vi "HDF5_Init_TC_Refs.vi"(5 "HDF5 file ref":T1 format="%.0x", 9 "File Exists?":bool, 11 "error in":errorcluster) -> (4 "TC_Refs":T2 {"TC13_Tamb_Inter" format="%.0x"; "TC12_Gen_Exhaust" format="%.0x"; "TC11_HVAC_Cond_Out" format="%.0x"; "TC10_HVAC_Cond_In" format="%.0x"; "TC9_LP2_Lo" format="%.0x"; "TC8_LP2_LoMid" format="%.0x"; "TC7_LP2_Mid" format="%.0x"; "TC6_LP2_MidHi" format="%.0x"; "TC5_LP2_Hi" format="%.0x"; "TC4_LP1_Lo" format="%.0x"; "TC3_LP1_LoMid" format="%.0x"; "TC2_LP1_Mid" format="%.0x"; "TC1_LP1_MidHi" format="%.0x"; "TC0_LP1_Hi" format="%.0x"; "TimeString_dset" format="%.0x"; "TimeStamp_dset" format="%.0x"; "Group_ref" format="%.0x"}, 6 "HDF5 file ref":T1 format="%.0x", 15 "error out":errorcluster)   [LabVIEW 2018]
doc: "Set up the HDF5 data structure and initialize the references for the Tone1, Tone2, Tone3, and Tone4 Groups and the datasets (tables) within each Group.\n\nData structure:\nTone1 (Group) \n Beac - cluster (Dataset)\n BeacZoom - 1024 element Double array (waveform) \n Cal - cluster\n CalZoom - 1024 element Double array (waveform) \nTone2\n Beac - cluster\n BeacZoom - 1024 element Double array (waveform) \n Cal - cluster\n CalZoom - 1024 element Double array (waveform) \nTone3\n Beac - cluster\n BeacZoom - 1024 element Double array (waveform) \n Cal - cluster\n CalZoom - 1024 element Double array (waveform) \nTone4\n Beac - cluster\n BeacZoom - 1024 element Double array (waveform) \n Cal - cluster\n CalZoom - 1024 element Double array (waveform)"
uses:
  <vilib>/addons/h5labview2/base/hid_t.ctl
  TC_Tone_refs.ctl
  lib_path_mod_20200519.vi
  <vilib>/addons/h5labview2/base/H5Equery.vi
  <vilib>/addons/h5labview2/attrib/H5Awrite.llb/H5Awrite.xnode
  <vilib>/addons/h5labview2/group/H5G.lvlib
  <vilib>/addons/h5labview2/dataset/H5D.lvlib
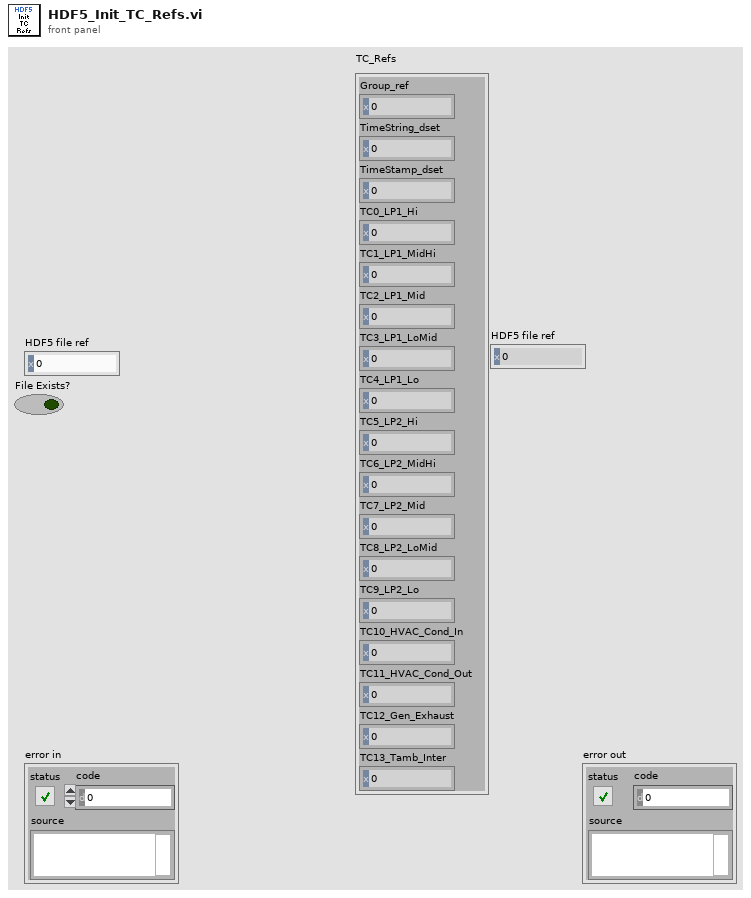
[diagram p1: front panel]
types:
  T1 = typedef "hid_t.ctl" = i32
  T2 = typedef "TC_Tone_refs.ctl" = cluster{"Group_ref":T1, "TimeString_dset":T1, "TimeStamp_dset":T1, "TC0_LP1_Hi":T1, "TC1_LP1_MidHi":T1, "TC2_LP1_Mid":T1, "TC3_LP1_LoMid":T1, "TC4_LP1_Lo":T1, "TC5_LP2_Hi":T1, "TC6_LP2_MidHi":T1, "TC7_LP2_Mid":T1, "TC8_LP2_LoMid":T1, "TC9_LP2_Lo":T1, "TC10_HVAC_Cond_In":T1, "TC11_HVAC_Cond_Out":T1, "TC12_Gen_Exhaust":T1, "TC13_Tamb_Inter":T1}
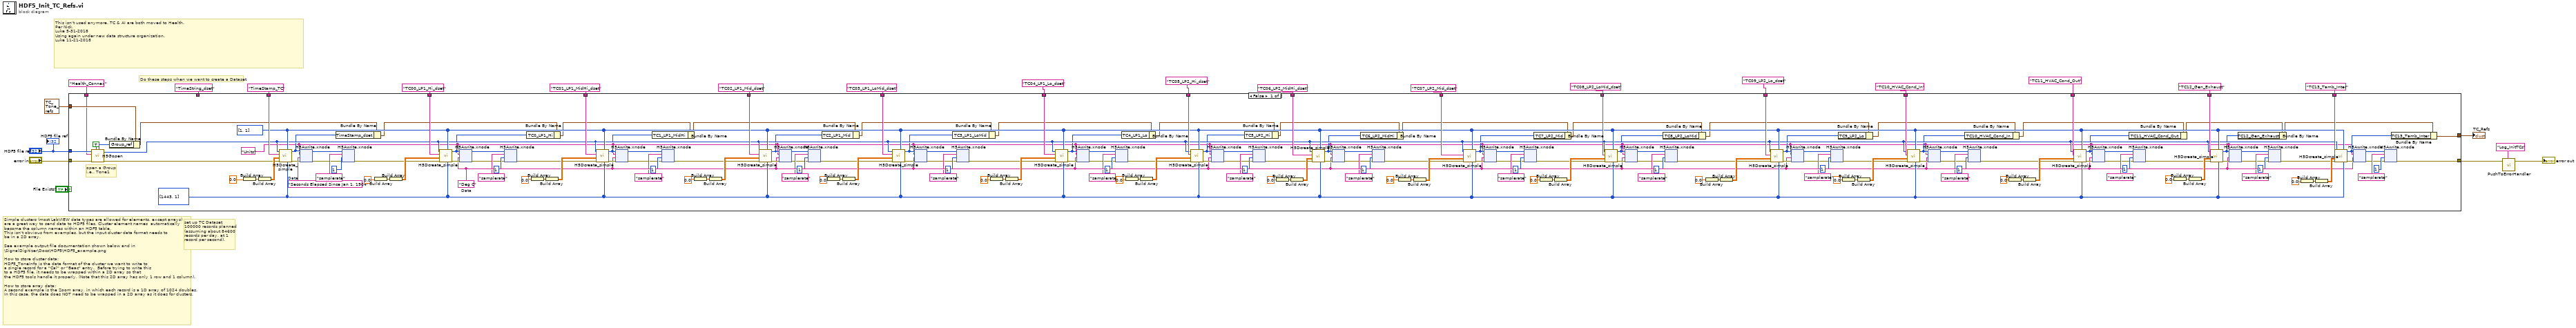
[diagram p0: block diagram]
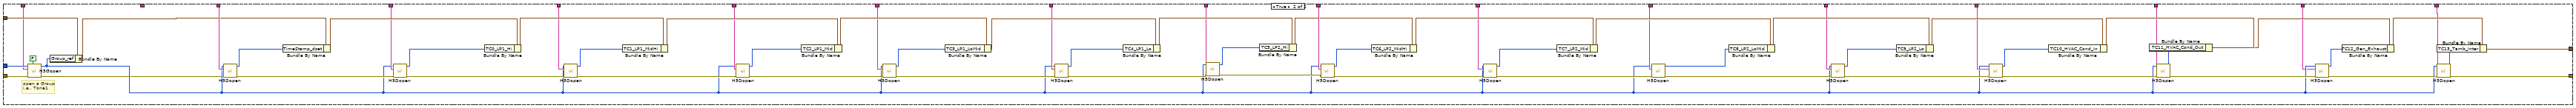
[diagram p2: hidden frame]
diagram:
  # "This isn't used anymore. TC & AI are both moved to Health.\nPer Nick.\nLuke 5-31-2018\nUsing again under new data structure organization.\nLuke 11-21-2018"
  # "Do these steps when we want to create a Dataset"
  # "set up TC Dataset\n100000 records planned\n(assuming about 84600\nrecords per day, at 1\nrecord per second)."
  # "Simple clusters (most LabVIEW data types are allowed for elements, except arrays) \nare a great way to send data to HDF5 files. Cluster element names  automatically\nbecome the column names within an HDF5 table.\nThis isn't obvious from examples, but the input cluster data format needs to \nbe in a 2D array.\n\nSee example output file documentation shown below and in\n\\SignalDigitizer\\Docs\\HDF5\\HDF5_example.png\n\nHow to store cluster data:\nHDF5_ToneInfo is the data format of the cluster we want to write to \na single record for a \"Cal\" or \"Beac\" entry.  Before trying to write this \nto a HDF5 file, it needs to be wrapped within a 2D array so that \nthe HDF5 tools handle it properly. (Note that this 2D array has only 1 row and 1 column).\n\nHow to store array data:\nA second example is the Zoom array, in which each record is a 1D array of 1024 doubles.\nIn this case, the data does NOT need to be wrapped in a 2D array as it does for clusters."
  n1 = case shown="False" "File Exists?" {
    tunnel: "error in" -> [w218 w856]
    tunnel: "HDF5 file ref" -> [w217 w855]
    tunnel: [w27 w792] -> w2
    tunnel: T2 {"Group_ref"=0, "TimeString_dset"=0, "TimeStamp_dset"=0, "TC0_LP1_Hi"=0, "TC1_LP1_MidHi"=0, "TC2_LP1_Mid"=0, "TC3_LP1_LoMid"=0, "TC4_LP1_Lo"=0, "TC5_LP2_Hi"=0, "TC6_LP2_MidHi"=0, "TC7_LP2_Mid"=0, "TC8_LP2_LoMid"=0, "TC9_LP2_Lo"=0, "TC10_HVAC_Cond_In"=0, "TC11_HVAC_Cond_Out"=0, "TC12_Gen_Exhaust"=0, "TC13_Tamb_Inter"=0} ("Cluster") -> [w215 w853]
    tunnel: [w153 w793] -> w22
    tunnel: "TimeString_dset" ("string") -> [_ _]
    tunnel: "TimeStamp_TC" ("string") -> [w214 w851]
    tunnel: "TC00_LP1_Hi_dset" ("string") -> [w208 w846]
    tunnel: "TC01_LP1_MidHi_dset" ("string") -> [w209 w837]
    tunnel: "TC02_LP1_Mid_dset" ("string") -> [w196 w836]
    tunnel: "TC03_LP1_LoMid_dset" ("string") -> [w197 w835]
    tunnel: "TC04_LP1_Lo_dset" ("string") -> [w203 w834]
    tunnel: "TC05_LP2_Hi_dset" ("string") -> [w202 w833]
    tunnel: "TC06_LP2_MidHi_dset" ("string") -> [w175 w821]
    tunnel: "TC07_LP2_Mid_dset" ("string") -> [w181 w819]
    tunnel: "TC08_LP2_LoMid_dset" ("string") -> [w180 w818]
    tunnel: "TC09_LP2_Lo_dset" ("string") -> [w191 w805]
    tunnel: "TC10_HVAC_Cond_In" ("string") -> [w190 w804]
    tunnel: "TC11_HVAC_Cond_Out" ("string") -> [w174 w803]
    tunnel: "TC12_Gen_Exhaust" ("string") -> [w173 w795]
    tunnel: "TC13_Tamb_Inter" ("string") -> [w157 w794]
    tunnel: "Health_Connex" ("name") -> [w103 w791]
    frame False {
      w104 = "Deg C"  # Data
      w132 = "Seconds Elapsed Since Jan 1, 1904"  # Data
      w105 = "Units" ("attrib name")
      w152 = u64[] [1, 1] ("chunk size")
      w154 = u64[] [1443, 1] ("max size")
      # "open a Group\ni.e., Tone1"
      n2 = call <vilib>:"H5Gopen.vi"("create? (F)"=TRUE, "error in (no error)"=w218, "name"=w103, "ref in"=w217) -> ("error out"=w102:errorcluster, "group out"=w149:T1)  [unwired: 6 in]
      n3 = Bundle By Name(cluster=w215, "Group_ref"=w149) -> (w101:T2)
      n4 = Build Array(0.0 ("TimeStamp")) -> (w212:dbl[])
      n5 = Build Array(w212) -> (w213:dbl[][])
      n6 = call <vilib>:"H5Dcreate_simple.vi"("max size"=w154, "chunk size"=w152, "error in (no error)"=w102, "type in"=w213, "name"=w214, "ref in"=w149) -> ("error out"=w136:errorcluster, "dset out"=w135:T1)  [unwired: 4 in]
      n7 = xnode "H5Awrite.xnode"("error in (no error)"=w136, "data"=w132, "attrib name"=w105, "ref in"=w135) -> ("error out"=w97:errorcluster, "ref out"=w98:i32)  [unwired: 3 in, 1 out]
      n8 = Bundle By Name(cluster=w101, "TimeStamp_dset"=w135) -> (w148:T2)
      n9 = xnode "H5Awrite.xnode"("error in (no error)"=w97, "data"=u32 1, "attrib name"="samplerate", "ref in"=w98) -> ("error out"=w96:errorcluster)  [unwired: 3 in, 2 out]
      n10 = Build Array(0.0) -> (w206:dbl[])
      n11 = Build Array(w206) -> (w207:dbl[][])
      n12 = call <vilib>:"H5Dcreate_simple.vi"("max size"=w154, "chunk size"=w152, "error in (no error)"=w96, "type in"=w207, "name"=w208, "ref in"=w149) -> ("error out"=w133:errorcluster, "dset out"=w134:T1)  [unwired: 4 in]
      n13 = xnode "H5Awrite.xnode"("error in (no error)"=w133, "data"=w104, "attrib name"=w105, "ref in"=w134) -> ("error out"=w92:errorcluster, "ref out"=w93:i32)  [unwired: 3 in, 1 out]
      n14 = xnode "H5Awrite.xnode"("error in (no error)"=w92, "data"=u32 1, "attrib name"="samplerate", "ref in"=w93) -> ("error out"=w91:errorcluster)  [unwired: 3 in, 2 out]
      n15 = Bundle By Name(cluster=w148, "TC0_LP1_Hi"=w134) -> (w147:T2)
      n16 = Build Array(0.0) -> (w211:dbl[])
      n17 = Build Array(w211) -> (w210:dbl[][])
      n18 = call <vilib>:"H5Dcreate_simple.vi"("max size"=w154, "chunk size"=w152, "error in (no error)"=w91, "type in"=w210, "name"=w209, "ref in"=w149) -> ("error out"=w131:errorcluster, "dset out"=w130:T1)  [unwired: 4 in]
      n19 = xnode "H5Awrite.xnode"("error in (no error)"=w131, "data"=w104, "attrib name"=w105, "ref in"=w130) -> ("error out"=w88:errorcluster, "ref out"=w87:i32)  [unwired: 3 in, 1 out]
      n20 = Bundle By Name(cluster=w147, "TC1_LP1_MidHi"=w130) -> (w146:T2)
      n21 = xnode "H5Awrite.xnode"("error in (no error)"=w88, "data"=u32 1, "attrib name"="samplerate", "ref in"=w87) -> ("error out"=w86:errorcluster)  [unwired: 3 in, 2 out]
      n22 = Build Array(0.0) -> (w194:dbl[])
      n23 = Build Array(w194) -> (w195:dbl[][])
      n24 = call <vilib>:"H5Dcreate_simple.vi"("max size"=w154, "chunk size"=w152, "error in (no error)"=w86, "type in"=w195, "name"=w196, "ref in"=w149) -> ("error out"=w128:errorcluster, "dset out"=w129:T1)  [unwired: 4 in]
      n25 = xnode "H5Awrite.xnode"("error in (no error)"=w128, "data"=w104, "attrib name"=w105, "ref in"=w129) -> ("error out"=w83:errorcluster, "ref out"=w82:i32)  [unwired: 3 in, 1 out]
      n26 = xnode "H5Awrite.xnode"("error in (no error)"=w83, "data"=u32 1, "attrib name"="samplerate", "ref in"=w82) -> ("error out"=w81:errorcluster)  [unwired: 3 in, 2 out]
      n27 = Bundle By Name(cluster=w146, "TC2_LP1_Mid"=w129) -> (w145:T2)
      n28 = Build Array(0.0) -> (w199:dbl[])
      n29 = Build Array(w199) -> (w198:dbl[][])
      n30 = call <vilib>:"H5Dcreate_simple.vi"("max size"=w154, "chunk size"=w152, "error in (no error)"=w81, "type in"=w198, "name"=w197, "ref in"=w149) -> ("error out"=w127:errorcluster, "dset out"=w126:T1)  [unwired: 4 in]
      n31 = xnode "H5Awrite.xnode"("error in (no error)"=w127, "data"=w104, "attrib name"=w105, "ref in"=w126) -> ("error out"=w78:errorcluster, "ref out"=w77:i32)  [unwired: 3 in, 1 out]
      n32 = Bundle By Name(cluster=w145, "TC3_LP1_LoMid"=w126) -> (w144:T2)
      n33 = xnode "H5Awrite.xnode"("error in (no error)"=w78, "data"=u32 1, "attrib name"="samplerate", "ref in"=w77) -> ("error out"=w76:errorcluster)  [unwired: 3 in, 2 out]
      n34 = Build Array(0.0) -> (w205:dbl[])
      n35 = Build Array(w205) -> (w204:dbl[][])
      n36 = call <vilib>:"H5Dcreate_simple.vi"("max size"=w154, "chunk size"=w152, "error in (no error)"=w76, "type in"=w204, "name"=w203, "ref in"=w149) -> ("error out"=w125:errorcluster, "dset out"=w121:T1)  [unwired: 4 in]
      n37 = xnode "H5Awrite.xnode"("error in (no error)"=w125, "data"=w104, "attrib name"=w105, "ref in"=w121) -> ("error out"=w73:errorcluster, "ref out"=w72:i32)  [unwired: 3 in, 1 out]
      n38 = xnode "H5Awrite.xnode"("error in (no error)"=w73, "data"=u32 1, "attrib name"="samplerate", "ref in"=w72) -> ("error out"=w71:errorcluster)  [unwired: 3 in, 2 out]
      n39 = Bundle By Name(cluster=w144, "TC4_LP1_Lo"=w121) -> (w143:T2)
      n40 = Build Array(0.0) -> (w200:dbl[])
      n41 = Build Array(w200) -> (w201:dbl[][])
      n42 = call <vilib>:"H5Dcreate_simple.vi"("max size"=w154, "chunk size"=w152, "error in (no error)"=w71, "type in"=w201, "name"=w202, "ref in"=w149) -> ("error out"=w124:errorcluster, "dset out"=w120:T1)  [unwired: 4 in]
      n43 = xnode "H5Awrite.xnode"("error in (no error)"=w124, "data"=w104, "attrib name"=w105, "ref in"=w120) -> ("error out"=w68:errorcluster, "ref out"=w67:i32)  [unwired: 3 in, 1 out]
      n44 = Bundle By Name(cluster=w143, "TC5_LP2_Hi"=w120) -> (w142:T2)
      n45 = xnode "H5Awrite.xnode"("error in (no error)"=w68, "data"=u32 1, "attrib name"="samplerate", "ref in"=w67) -> ("error out"=w66:errorcluster)  [unwired: 3 in, 2 out]
      n46 = Build Array(0.0) -> (w177:dbl[])
      n47 = Build Array(w177) -> (w176:dbl[][])
      n48 = call <vilib>:"H5Dcreate_simple.vi"("max size"=w154, "chunk size"=w152, "error in (no error)"=w66, "type in"=w176, "name"=w175, "ref in"=w149) -> ("error out"=w123:errorcluster, "dset out"=w119:T1)  [unwired: 4 in]
      n49 = xnode "H5Awrite.xnode"("error in (no error)"=w123, "data"=w104, "attrib name"=w105, "ref in"=w119) -> ("error out"=w63:errorcluster, "ref out"=w62:i32)  [unwired: 3 in, 1 out]
      n50 = Bundle By Name(cluster=w142, "TC6_LP2_MidHi"=w119) -> (w141:T2)
      n51 = xnode "H5Awrite.xnode"("error in (no error)"=w63, "data"=u32 1, "attrib name"="samplerate", "ref in"=w62) -> ("error out"=w61:errorcluster)  [unwired: 3 in, 2 out]
      n52 = Build Array(0.0) -> (w183:dbl[])
      n53 = Build Array(w183) -> (w182:dbl[][])
      n54 = call <vilib>:"H5Dcreate_simple.vi"("max size"=w154, "chunk size"=w152, "error in (no error)"=w61, "type in"=w182, "name"=w181, "ref in"=w149) -> ("error out"=w122:errorcluster, "dset out"=w118:T1)  [unwired: 4 in]
      n55 = xnode "H5Awrite.xnode"("error in (no error)"=w122, "data"=w104, "attrib name"=w105, "ref in"=w118) -> ("error out"=w58:errorcluster, "ref out"=w57:i32)  [unwired: 3 in, 1 out]
      n56 = xnode "H5Awrite.xnode"("error in (no error)"=w58, "data"=u32 1, "attrib name"="samplerate", "ref in"=w57) -> ("error out"=w56:errorcluster)  [unwired: 3 in, 2 out]
      n57 = Bundle By Name(cluster=w141, "TC7_LP2_Mid"=w118) -> (w140:T2)
      n58 = Build Array(0.0) -> (w178:dbl[])
      n59 = Build Array(w178) -> (w179:dbl[][])
      n60 = call <vilib>:"H5Dcreate_simple.vi"("max size"=w154, "chunk size"=w152, "error in (no error)"=w56, "type in"=w179, "name"=w180, "ref in"=w149) -> ("error out"=w117:errorcluster, "dset out"=w113:T1)  [unwired: 4 in]
      n61 = xnode "H5Awrite.xnode"("error in (no error)"=w117, "data"=w104, "attrib name"=w105, "ref in"=w113) -> ("error out"=w53:errorcluster, "ref out"=w52:i32)  [unwired: 3 in, 1 out]
      n62 = Bundle By Name(cluster=w140, "TC8_LP2_LoMid"=w113) -> (w139:T2)
      n63 = xnode "H5Awrite.xnode"("error in (no error)"=w53, "data"=u32 1, "attrib name"="samplerate", "ref in"=w52) -> ("error out"=w51:errorcluster)  [unwired: 3 in, 2 out]
      n64 = Build Array(0.0) -> (w193:dbl[])
      n65 = Build Array(w193) -> (w192:dbl[][])
      n66 = call <vilib>:"H5Dcreate_simple.vi"("max size"=w154, "chunk size"=w152, "error in (no error)"=w51, "type in"=w192, "name"=w191, "ref in"=w149) -> ("error out"=w116:errorcluster, "dset out"=w112:T1)  [unwired: 4 in]
      n67 = xnode "H5Awrite.xnode"("error in (no error)"=w116, "data"=w104, "attrib name"=w105, "ref in"=w112) -> ("error out"=w48:errorcluster, "ref out"=w47:i32)  [unwired: 3 in, 1 out]
      n68 = xnode "H5Awrite.xnode"("error in (no error)"=w48, "data"=u32 1, "attrib name"="samplerate", "ref in"=w47) -> ("error out"=w46:errorcluster)  [unwired: 3 in, 2 out]
      n69 = Bundle By Name(cluster=w139, "TC9_LP2_Lo"=w112) -> (w138:T2)
      n70 = Build Array(0.0) -> (w188:dbl[])
      n71 = Build Array(w188) -> (w189:dbl[][])
      n72 = call <vilib>:"H5Dcreate_simple.vi"("max size"=w154, "chunk size"=w152, "error in (no error)"=w46, "type in"=w189, "name"=w190, "ref in"=w149) -> ("error out"=w115:errorcluster, "dset out"=w111:T1)  [unwired: 4 in]
      n73 = xnode "H5Awrite.xnode"("error in (no error)"=w115, "data"=w104, "attrib name"=w105, "ref in"=w111) -> ("error out"=w43:errorcluster, "ref out"=w42:i32)  [unwired: 3 in, 1 out]
      n74 = Bundle By Name(cluster=w138, "TC10_HVAC_Cond_In"=w111) -> (w137:T2)
      n75 = xnode "H5Awrite.xnode"("error in (no error)"=w43, "data"=u32 1, "attrib name"="samplerate", "ref in"=w42) -> ("error out"=w41:errorcluster)  [unwired: 3 in, 2 out]
      n76 = Build Array(0.0) -> (w184:dbl[])
      n77 = Build Array(w184) -> (w185:dbl[][])
      n78 = call <vilib>:"H5Dcreate_simple.vi"("max size"=w154, "chunk size"=w152, "error in (no error)"=w41, "type in"=w185, "name"=w174, "ref in"=w149) -> ("error out"=w114:errorcluster, "dset out"=w110:T1)  [unwired: 4 in]
      n79 = xnode "H5Awrite.xnode"("error in (no error)"=w114, "data"=w104, "attrib name"=w105, "ref in"=w110) -> ("error out"=w38:errorcluster, "ref out"=w37:i32)  [unwired: 3 in, 1 out]
      n80 = Bundle By Name(cluster=w137, "TC11_HVAC_Cond_Out"=w110) -> (w151:T2)
      n81 = xnode "H5Awrite.xnode"("error in (no error)"=w38, "data"=u32 1, "attrib name"="samplerate", "ref in"=w37) -> ("error out"=w36:errorcluster)  [unwired: 3 in, 2 out]
      n82 = Build Array(0.0) -> (w187:dbl[])
      n83 = Build Array(w187) -> (w186:dbl[][])
      n84 = call <vilib>:"H5Dcreate_simple.vi"("max size"=w154, "chunk size"=w152, "error in (no error)"=w36, "type in"=w186, "name"=w173, "ref in"=w149) -> ("error out"=w109:errorcluster, "dset out"=w106:T1)  [unwired: 4 in]
      n85 = xnode "H5Awrite.xnode"("error in (no error)"=w109, "data"=w104, "attrib name"=w105, "ref in"=w106) -> ("error out"=w33:errorcluster, "ref out"=w32:i32)  [unwired: 3 in, 1 out]
      n86 = Bundle By Name(cluster=w151, "TC12_Gen_Exhaust"=w106) -> (w150:T2)
      n87 = xnode "H5Awrite.xnode"("error in (no error)"=w33, "data"=u32 1, "attrib name"="samplerate", "ref in"=w32) -> ("error out"=w31:errorcluster)  [unwired: 3 in, 2 out]
      n88 = Build Array(0.0) -> (w155:dbl[])
      n89 = Build Array(w155) -> (w156:dbl[][])
      n90 = call <vilib>:"H5Dcreate_simple.vi"("max size"=w154, "chunk size"=w152, "error in (no error)"=w31, "type in"=w156, "name"=w157, "ref in"=w149) -> ("error out"=w108:errorcluster, "dset out"=w107:T1)  [unwired: 4 in]
      n91 = xnode "H5Awrite.xnode"("error in (no error)"=w108, "data"=w104, "attrib name"=w105, "ref in"=w107) -> ("error out"=w28:errorcluster, "ref out"=w26:i32)  [unwired: 3 in, 1 out]
      n92 = xnode "H5Awrite.xnode"("error in (no error)"=w28, "data"=u32 1, "attrib name"="samplerate", "ref in"=w26) -> ("error out"=w27:errorcluster)  [unwired: 3 in, 2 out]
      n93 = Bundle By Name(cluster=w150, "TC13_Tamb_Inter"=w107) -> (w153:T2)
    }
    frame True {
      # "open a Group\ni.e., Tone1"
      n94 = call <vilib>:"H5Gopen.vi"("create? (F)"=FALSE, "error in (no error)"=w856, "name"=w791, "ref in"=w855) -> ("error out"=w789:errorcluster, "group out"=w796:T1)  [unwired: 6 in]
      n95 = Bundle By Name(cluster=w853, "Group_ref"=w796) -> (w790:T2)
      n96 = call <vilib>:"H5Dopen.vi"("error in (no error)"=w789, "name"=w851, "loc in"=w796) -> ("error out"=w817:errorcluster, "dset out"=w852:T1)  [unwired: 7 in]
      n97 = Bundle By Name(cluster=w790, "TimeStamp_dset"=w852) -> (w847:T2)
      n98 = call <vilib>:"H5Dopen.vi"("error in (no error)"=w817, "name"=w846, "loc in"=w796) -> ("error out"=w816:errorcluster, "dset out"=w848:T1)  [unwired: 7 in]
      n99 = Bundle By Name(cluster=w847, "TC0_LP1_Hi"=w848) -> (w850:T2)
      n100 = call <vilib>:"H5Dopen.vi"("error in (no error)"=w816, "name"=w837, "loc in"=w796) -> ("error out"=w815:errorcluster, "dset out"=w849:T1)  [unwired: 7 in]
      n101 = Bundle By Name(cluster=w850, "TC1_LP1_MidHi"=w849) -> (w838:T2)
      n102 = call <vilib>:"H5Dopen.vi"("error in (no error)"=w815, "name"=w836, "loc in"=w796) -> ("error out"=w814:errorcluster, "dset out"=w839:T1)  [unwired: 7 in]
      n103 = Bundle By Name(cluster=w838, "TC2_LP1_Mid"=w839) -> (w841:T2)
      n104 = call <vilib>:"H5Dopen.vi"("error in (no error)"=w814, "name"=w835, "loc in"=w796) -> ("error out"=w813:errorcluster, "dset out"=w840:T1)  [unwired: 7 in]
      n105 = Bundle By Name(cluster=w841, "TC3_LP1_LoMid"=w840) -> (w845:T2)
      n106 = call <vilib>:"H5Dopen.vi"("error in (no error)"=w813, "name"=w834, "loc in"=w796) -> ("error out"=w812:errorcluster, "dset out"=w844:T1)  [unwired: 7 in]
      n107 = Bundle By Name(cluster=w845, "TC4_LP1_Lo"=w844) -> (w842:T2)
      n108 = call <vilib>:"H5Dopen.vi"("error in (no error)"=w812, "name"=w833, "loc in"=w796) -> ("error out"=w811:errorcluster, "dset out"=w843:T1)  [unwired: 7 in]
      n109 = Bundle By Name(cluster=w842, "TC5_LP2_Hi"=w843) -> (w820:T2)
      n110 = call <vilib>:"H5Dopen.vi"("error in (no error)"=w811, "name"=w821, "loc in"=w796) -> ("error out"=w810:errorcluster, "dset out"=w824:T1)  [unwired: 7 in]
      n111 = Bundle By Name(cluster=w820, "TC6_LP2_MidHi"=w824) -> (w822:T2)
      n112 = call <vilib>:"H5Dopen.vi"("error in (no error)"=w810, "name"=w819, "loc in"=w796) -> ("error out"=w809:errorcluster, "dset out"=w823:T1)  [unwired: 7 in]
      n113 = Bundle By Name(cluster=w822, "TC7_LP2_Mid"=w823) -> (w832:T2)
      n114 = call <vilib>:"H5Dopen.vi"("error in (no error)"=w809, "name"=w818, "loc in"=w796) -> ("error out"=w808:errorcluster, "dset out"=w831:T1)  [unwired: 7 in]
      n115 = Bundle By Name(cluster=w832, "TC8_LP2_LoMid"=w831) -> (w829:T2)
      n116 = call <vilib>:"H5Dopen.vi"("error in (no error)"=w808, "name"=w805, "loc in"=w796) -> ("error out"=w807:errorcluster, "dset out"=w830:T1)  [unwired: 7 in]
      n117 = Bundle By Name(cluster=w829, "TC9_LP2_Lo"=w830) -> (w825:T2)
      n118 = call <vilib>:"H5Dopen.vi"("error in (no error)"=w807, "name"=w804, "loc in"=w796) -> ("error out"=w806:errorcluster, "dset out"=w826:T1)  [unwired: 7 in]
      n119 = Bundle By Name(cluster=w825, "TC10_HVAC_Cond_In"=w826) -> (w828:T2)
      n120 = call <vilib>:"H5Dopen.vi"("error in (no error)"=w806, "name"=w803, "loc in"=w796) -> ("error out"=w797:errorcluster, "dset out"=w827:T1)  [unwired: 7 in]
      n121 = Bundle By Name(cluster=w828, "TC11_HVAC_Cond_Out"=w827) -> (w798:T2)
      n122 = call <vilib>:"H5Dopen.vi"("error in (no error)"=w797, "name"=w795, "loc in"=w796) -> ("error out"=w802:errorcluster, "dset out"=w801:T1)  [unwired: 7 in]
      n123 = Bundle By Name(cluster=w798, "TC12_Gen_Exhaust"=w801) -> (w799:T2)
      n124 = call <vilib>:"H5Dopen.vi"("error in (no error)"=w802, "name"=w794, "loc in"=w796) -> ("error out"=w792:errorcluster, "dset out"=w800:T1)  [unwired: 7 in]
      n125 = Bundle By Name(cluster=w799, "TC13_Tamb_Inter"=w800) -> (w793:T2)
    }
  }
  "TC_Refs" <- w22
  n126 = call "PushToErrorHandler.vi"("ErrorIn"=w2, "ErrorLocation"="Log_InitTCs") -> ("ErrorOut"=→"error out":errorcluster)  [unwired: 5 in]
  "HDF5 file ref" <- "HDF5 file ref"
